vi "Compute_Anomaly_Map(CuLab).vi"(8 "error in":errorcluster, 9 "Gaussian Blur":T1={"Kernel_Size"=33, "sigma"=4.0}, 10 "input img size":i32[](array[numeric])=[224, 224], 11 "patch scores [bs,w,h]":refnum<class "T3D_SGL.lvclass">) -> (0 "error out":errorcluster, 3 "anomaly map":refnum<class "T3D_SGL.lvclass">)   [LabVIEW 2020]
uses:
  API/Controls/Gaussian_Blur.ctl
  <vilib>/Ngene/CuLab - GPU Accelerated Toolkit/Toolkit/Low_Level/Tensor_Classes/T_Children/T3D/T3D_Children/T3D_SGL/T3D_SGL.lvclass
  C:/Program Files/National Instruments/LabVIEW 2020/vi.lib/Ngene/CuLab - GPU Accelerated Toolkit/Toolkit/Low_Level/Tensor_Classes/T_Children/T3D/T3D.lvclass
  <vilib>/Ngene/CuLab - GPU Accelerated Toolkit/Toolkit/API/Computer Vision/Vision Utilities/Image Manipulation/Resample/Controls/Interpolation_Enum.ctl
  <vilib>/Ngene/CuLab - GPU Accelerated Toolkit/Toolkit/Low_Level/Tensor_Classes/T_Children/T2D/Controls/T2D_Dims.ctl
  <vilib>/Ngene/CuLab - GPU Accelerated Toolkit/Toolkit/Low_Level/Tensor_Classes/T_Children/T2D/T2D_Children/T2D_SGL/T2D_SGL.lvclass
  C:/Program Files/National Instruments/LabVIEW 2020/vi.lib/Ngene/CuLab - GPU Accelerated Toolkit/Toolkit/Low_Level/Tensor_Classes/T_Children/T2D/T2D.lvclass
  C:/Program Files/National Instruments/LabVIEW 2020/vi.lib/Ngene/CuLab - GPU Accelerated Toolkit/Toolkit/Low_Level/Tensor_Classes/Tensor.lvclass
  <vilib>/Ngene/CuLab - GPU Accelerated Toolkit/Toolkit/Low_Level/Tensor_Classes/T_Children/T2D/Controls/T2D_Indices.ctl
  702c6057-13e7-4734-9589-5e72ce7024bb.vi
  <vilib>/Ngene/Deep Learning Toolkit/Toolkit/NN_Layers/Layers/Input/subVIs/Augmentation/Blur/SubVI/Gauss_Function.vi
  <vilib>/Ngene/CuLab - GPU Accelerated Toolkit/Toolkit/API/Computer Vision/Vision Utilities/Image Manipulation/Resample/CU_CV_Resample_T2D_SGL_batch.vi
  <vilib>/Ngene/CuLab - GPU Accelerated Toolkit/Toolkit/API/Array/Array Size/CU_Array_Size_T3D.vi
  <vilib>/Ngene/CuLab - GPU Accelerated Toolkit/Toolkit/Low_Level/Tensor_Classes/T_Children/T2D/T2D_Children/T2D_SGL/Create_Push.vi
  <vilib>/Ngene/CuLab - GPU Accelerated Toolkit/Toolkit/API/Array/Index Array Subset/T3D/CU_Index_Array_Subset_T3D_SGL.vi
  <vilib>/Ngene/CuLab - GPU Accelerated Toolkit/Toolkit/API/Signal Processing/Signal Operation/Convolution/T2D/CU_Convolution_T2D_SGL.vi
  <vilib>/Ngene/CuLab - GPU Accelerated Toolkit/Toolkit/API/Array/Replace Array Subset (API)/CU_Replace_Array_Subset_2D_2D/CU_Replace_Array_Subset_2D_2D_SGL.vi
  <vilib>/Ngene/CuLab - GPU Accelerated Toolkit/Toolkit/API/Array/Reshape Array  (API)/CU_Reshape_to_T3D/T2D/CU_Reshape_to_T3D_(T2D_SGL).vi
  <vilib>/Ngene/Deep Learning Toolkit/Toolkit/Deep_Learning_Toolkit_by_Ngene.lvlib
  <vilib>/Ngene/CuLab - GPU Accelerated Toolkit/Toolkit/CuLab.lvlib
  <vilib>/Ngene/CuLab - GPU Accelerated Toolkit/Toolkit/Low_Level/Tensor_Classes/Tensor.lvclass
  <vilib>/Ngene/CuLab - GPU Accelerated Toolkit/Toolkit/Low_Level/Tensor_Classes/T_Children/T0D/T0D_Children/T0D_CDB/T0D_CDB.lvclass
  C:/Program Files/National Instruments/LabVIEW 2020/vi.lib/Ngene/CuLab - GPU Accelerated Toolkit/Toolkit/Low_Level/Tensor_Classes/T_Children/T3D/T3D_Children/T3D_SGL/T3D_SGL.lvclass
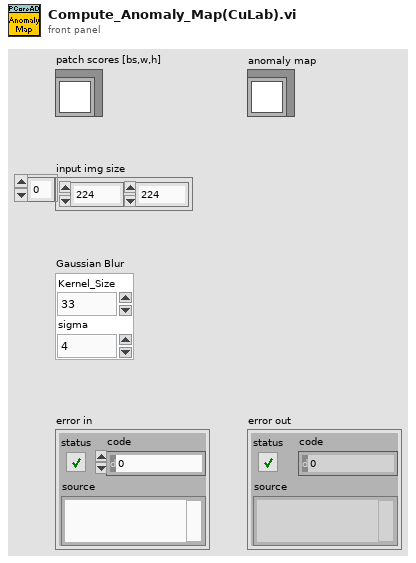
[diagram p1: front panel]
types:
  T1 = typedef "Gaussian_Blur.ctl" = cluster{"Kernel_Size":i32, "sigma":sgl}
  T2 = typedef "CuLab.lvlib/Interpolation_Enum.ctl" = enum32{"Zero Order", "Bi-Linear", "Quadratic"}
  T3 = typedef "CuLab.lvlib/T2D_Dims.ctl" = cluster{"H":i32, "W":i32}
  T4 = typedef "CuLab.lvlib/T2D_Indices.ctl" = cluster{"i":i32, "j":i32}
  T5 = typedef "CuLab.lvlib/T3D_Dims.ctl" = cluster{"C ":i32, "H":i32, "W":i32}
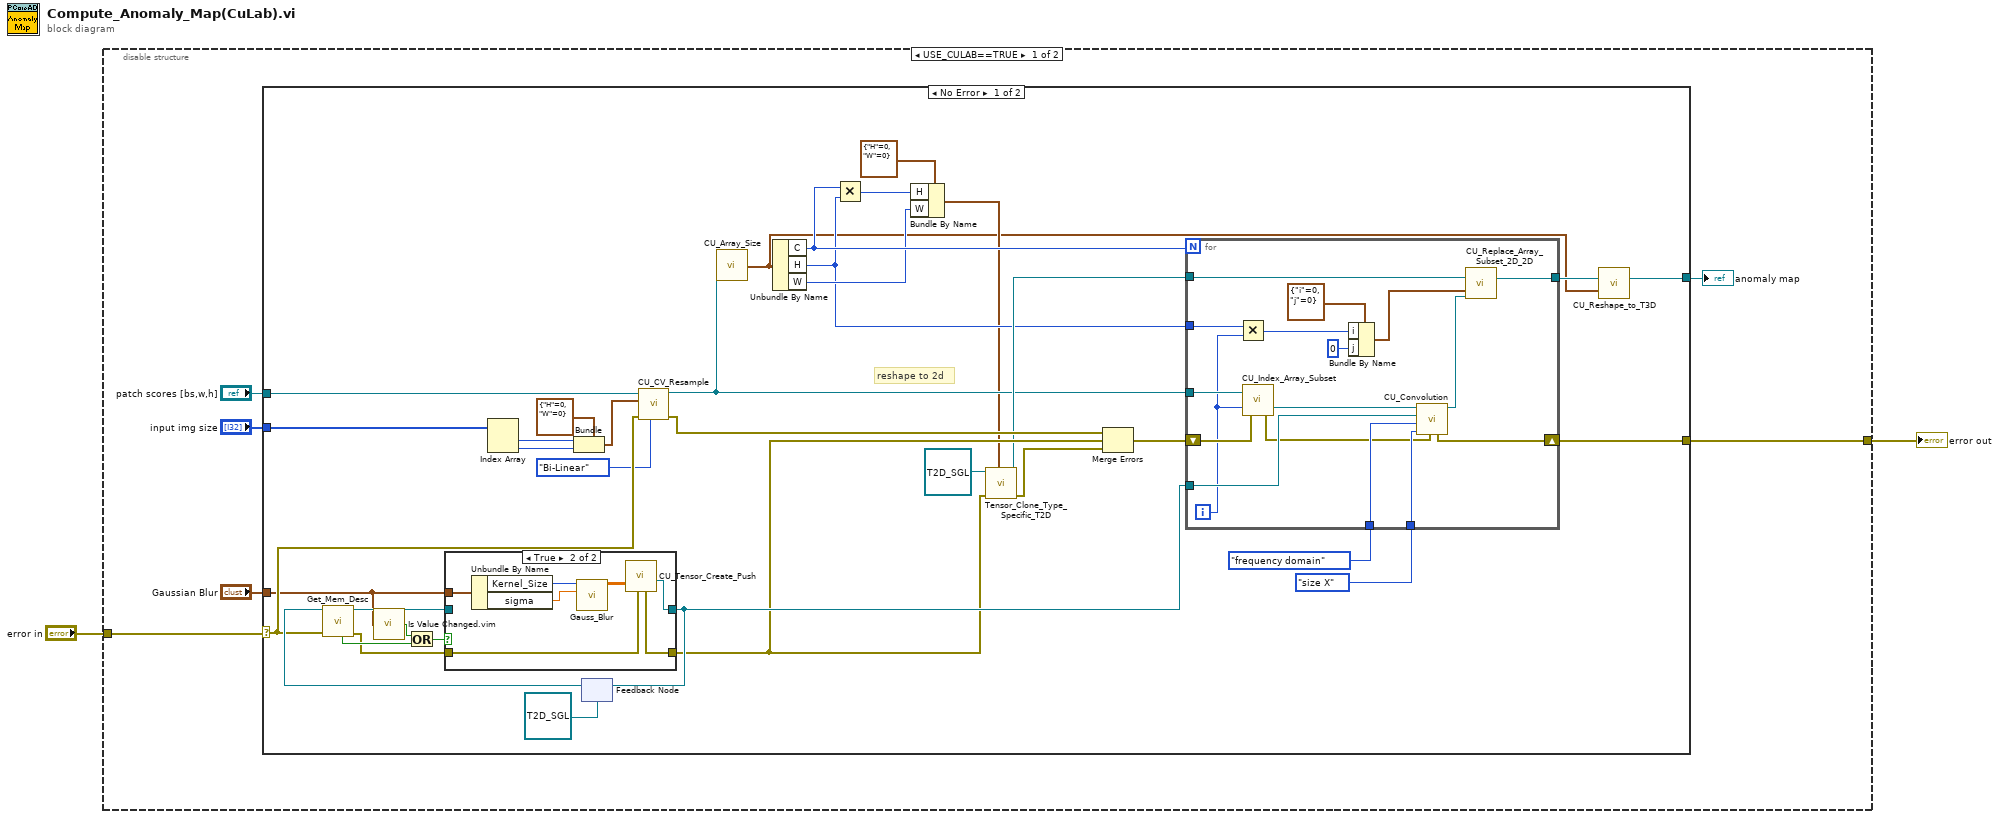
[diagram p0: block diagram]
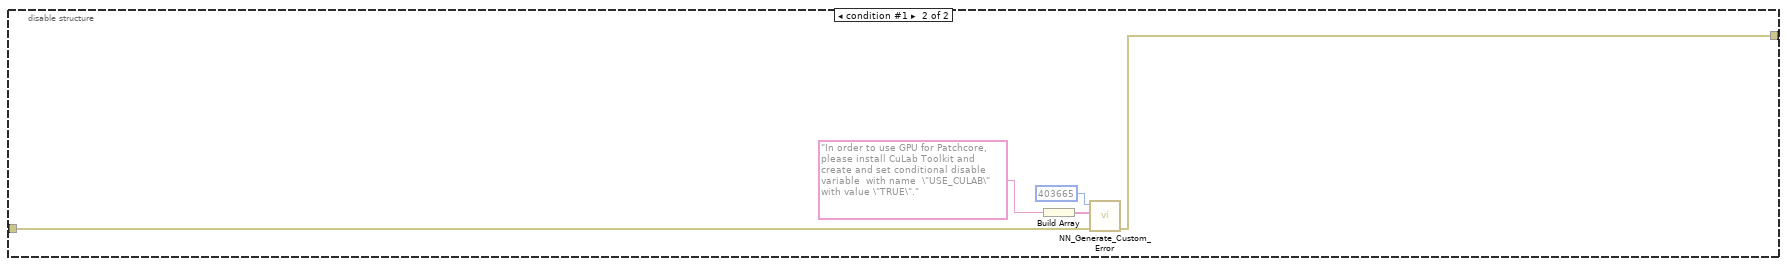
[diagram p4: hidden frame]
diagram:
  n1 = disable-structure shown="USE_CULAB==TRUE" {
    disable-tunnel: [w4 w72] -> w2
    disable-tunnel: "error in" -> [w3 w73]
    frame condition #0 (active) {
      n2 = case shown="No Error" w3 {
        selector: w3 -> [w35 w71]
        tunnel: "input img size" -> [w43 _]
        tunnel: "patch scores [bs,w,h]" -> [w44 _]
        tunnel: [w33 w71] -> w4
        tunnel: "Gaussian Blur" -> [w9 _]
        tunnel: [w15 _] -> w5
        frame No Error {
          # "reshape to 2d"
          n3 = call "Is Value Changed.vim"("value"=w9) -> ("changed or first call?"=w36:bool)
          n4 = Index Array(array=w43) -> (element #1=w12:i32, element #2=w13:i32)  [unwired: 2 in]
          n5 = Bundle(cluster=T3 {"H"=0, "W"=0} ("Dest Resoltuion"), "H"=w12, "W"=w13) -> (w10:T3)
          n6 = feedback #1(refnum<class "T2D_SGL.lvclass"> refnum ("T2D_SGL out")) -> (w41:refnum<class "T2D_SGL.lvclass">)
          n7 = call <vilib>:"Get_Mem_Desc.vi"("error in (no error)"=w35, "Tensor in"=w41) -> ("error out"=w34:errorcluster, "Tensor out"=w37:refnum<class "T2D_SGL.lvclass">, "Empty?"=w40:bool)  [unwired: 5 in, 2 out]
          n8 = Or(x=w36, y=w40) -> (x .or. y?=w39:bool)
          n9 = case shown="True" w39 {
            tunnel: w9 -> [_ w70]
            tunnel: [w63 w67] -> w42
            tunnel: w37 -> [w63 _]
            tunnel: w34 -> [w62 w65]
            tunnel: [w62 w64] -> w27
            frame False {
            }
            frame True {
              n10 = Unbundle By Name(w70) -> ("Kernel_Size"=w69:i32, "sigma"=w68:sgl)
              n11 = call <vilib>:"Gauss_Blur.vi"("sigma"=w68, "Kernel_Size"=w69) -> ("Kernel"=w66:sgl[][])  [unwired: 9 in]
              n12 = call-poly <vilib>:"CU_Tensor_Create_Push.vi"("error in (no error)"=w65, "CPU_Data_2D_SGL"=w66) -> ("T2D_SGL out"=w67:refnum<class "T2D_SGL.lvclass">, "error out"=w64:errorcluster)  [unwired: 8 in]
            }
          }
          n13 = feedback-in #1(w42) -> ()
          n14 = call-poly <vilib>:"CU_CV_Resample.vi"("Interpolation Type"=Interpolation_Enum."Bi-Linear", "error in (no error)"=w35, "Dest Resoltuion"=w10, "Src"=w44) -> ("error out"=w30:errorcluster, "Dest out"=w19:refnum<class "T3D_SGL.lvclass">)  [unwired: 6 in]
          n15 = call-poly <vilib>:"CU_Array_Size.vi"("Tensor"=w19) -> ("T3D_Dims"=w16:T5)  [unwired: 14 in]
          n16 = Unbundle By Name(w16) -> ("C"=w24:i32, "H"=w20:i32, "W"=w22:i32)
          n17 = Multiply(x=w24, y=w20) -> (x*y=w23:i32)
          n18 = Bundle By Name(cluster=T3 {"H"=0, "W"=0} ("Dest_Tensor_Dims"), "H"=w23, "W"=w22) -> (w18:T3)
          n19 = call <vilib>:"Tensor_Clone_Type_Specific_T2D.vi"("Dest_Tensor_Dims"=w18, "error in (no error)"=w27, "Dest_Tensor"=refnum<class "T2D_SGL.lvclass"> refnum ("initialized Tensor")) -> ("error out"=w26:errorcluster, "Dest_Tensor out"=w21:refnum<class "T2D_SGL.lvclass">)  [unwired: 7 in]
          n20 = Merge Errors(w30, w27, w26) -> (w28:errorcluster)
          n21 = for {
            N: w24 -> [_]
            tunnel: w19 -> [w54]
            tunnel: enum32{"direct", "frequency domain"}."frequency domain" ("algorithm") -> [w58]
            tunnel: enum32{"full", "size X", "compact"}."size X" ("output size") -> [w57]
            shift-right: [w59] -> w33
            shift-left: w28 -> [w56]
            tunnel: w42 -> [w60]
            tunnel: w21 -> [w53]
            tunnel: w20 -> [w48]
            tunnel: [w45] -> w17
            i -> [w50]
            n22 = Multiply(x=w48, y=w50) -> (x*y=w49:i32)
            n23 = call-poly <vilib>:"CU_Index_Array_Subset.vi"("Tensor in"=w54, "Channel"=w50, "error in (no error)"=w56) -> ("error out"=w55:errorcluster, "Sub Tensor"=w61:refnum<class "T2D_SGL.lvclass">)  [unwired: 15 in]
            n24 = Bundle By Name(cluster=T4 {"i"=0, "j"=0} ("Indices"), "i"=w49, "j"=0) -> (w47:T4)
            n25 = call-poly <vilib>:"CU_Convolution.vi"("error in"=w55, "output size"=w57, "algorithm"=w58, "Y"=w60, "X"=w61) -> ("X * Y"=w46:refnum<class "T2D_SGL.lvclass">, "error out"=w59:errorcluster)  [unwired: 5 in]
            n26 = call-poly <vilib>:"CU_Replace_Array_Subset_2D_2D.vi"("Tensor in"=w53, "Indices"=w47, "Sub Tensor"=w46) -> ("Tensor Out"=w45:refnum<class "T2D_SGL.lvclass">)  [unwired: 11 in, 1 out]
          }
          n27 = call-poly <vilib>:"CU_Reshape_to_T3D.vi"("Tensor in"=w17, "Dest Dims"=w16) -> ("Dest out"=w15:refnum<class "T3D_SGL.lvclass">)  [unwired: 12 in, 1 out]
        }
        frame Error {
        }
      }
      "anomaly map" <- w5
    }
    frame condition #1 {
      n28 = Build Array("In order to use GPU for Patchcore, please install CuLab Toolkit and create and set conditional disable variable  with name  \"USE_CULAB\" with value \"TRUE\"." ("Message")) -> (w75:string[])
      n29 = call <vilib>:"NN_Generate_Custom_Error.vi"("error in (no error)"=w73, "Message"=w75, "Error_code"=403665) -> ("error out"=w72:errorcluster)  [unwired: 8 in]
    }
  }
  "error out" <- w2
